vi "RegisterMap_ RegMap Sort.vi"(8 "error in (no error)":errorcluster, 10 "Register RegMap Data":string[][](array[string]), 11 "Register Data IN":T1[](array[typedef]) {"Base" format="%.0x"; "Item Count" format="%.0x"; "Value" format="%.0x"; "RegMap"."Mask" format="%.0x"; "Default" format="%.0x"; "Register" format="%.0x"}) -> (0 "error out":errorcluster, 3 "Register Data OUT":T1[](array[typedef]) {"Base" format="%.0x"; "Item Count" format="%.0x"; "Value" format="%.0x"; "RegMap"."Mask" format="%.0x"; "Default" format="%.0x"; "Register" format="%.0x"})   [LabVIEW 2010]
doc: "This VI sorts the RegMap data that was split into components and updates the Register Map array with the information.\n\nInputs:\nAMC Register Data IN - (cluster[]) array containing register map data\nRegister RegMap Data - (str[]) string array containing the register format for each register\nerror in - error input cluster\n\nOutputs:\nAMC Register Data OUT - (cluster[]) updated input array\nBit Count Verify Array - (U16) array displaying counted length of each register (should all be equal to the register length/size) (LOCAL only)\nAll Registers Equal Length? - (bool) TRUE = all registers are equal length (LOCAL only)\nerror out - error output cluster"
uses:
  TYP_ADSxxxx Register.ctl
  TYP_RegMap Item.ctl
panel:
  out "All Register Equal Length?":bool
  out "Bit Count Verify Array":u16[](array[numeric])
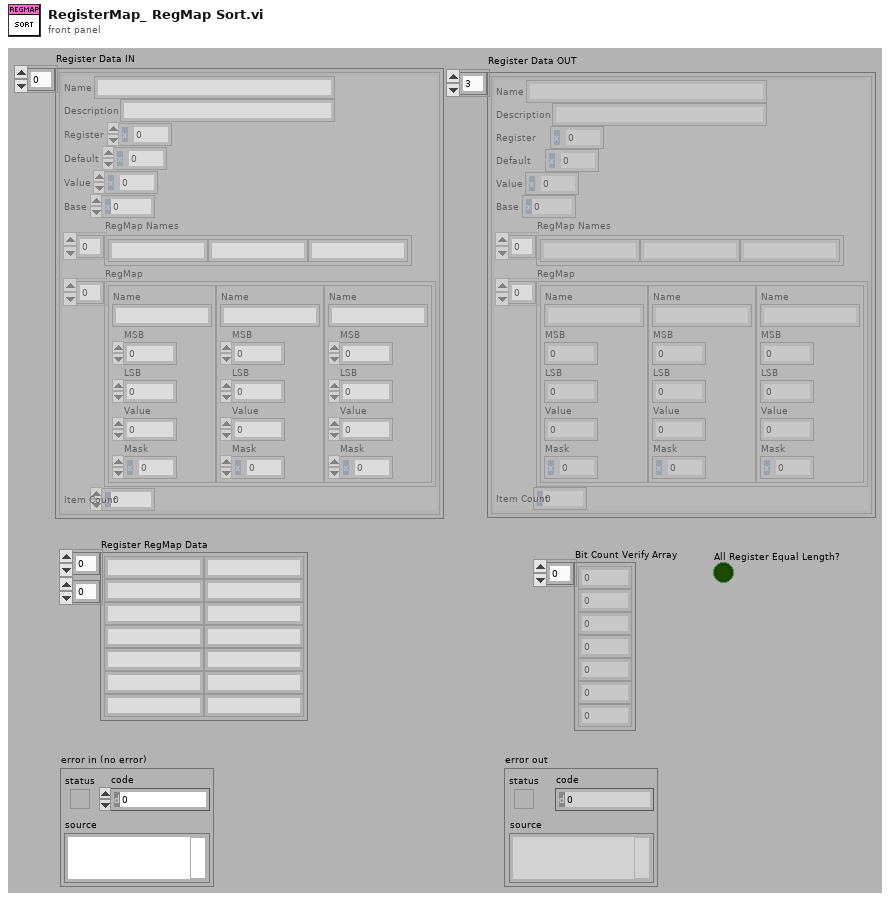
[diagram p1: front panel]
types:
  T1 = typedef "TYP_ADSxxxx Register.ctl" = cluster{"Name":string, "Description":string, "Register":u16, "Default":u16, "Value":u16, "Base":u16, "RegMap Names":string[], "RegMap":T2[], "Item Count":u8}
  T2 = typedef "TYP_RegMap Item.ctl" = cluster{"Name":string, "MSB":u16, "LSB":u16, "Value":u16, "Mask":u16}
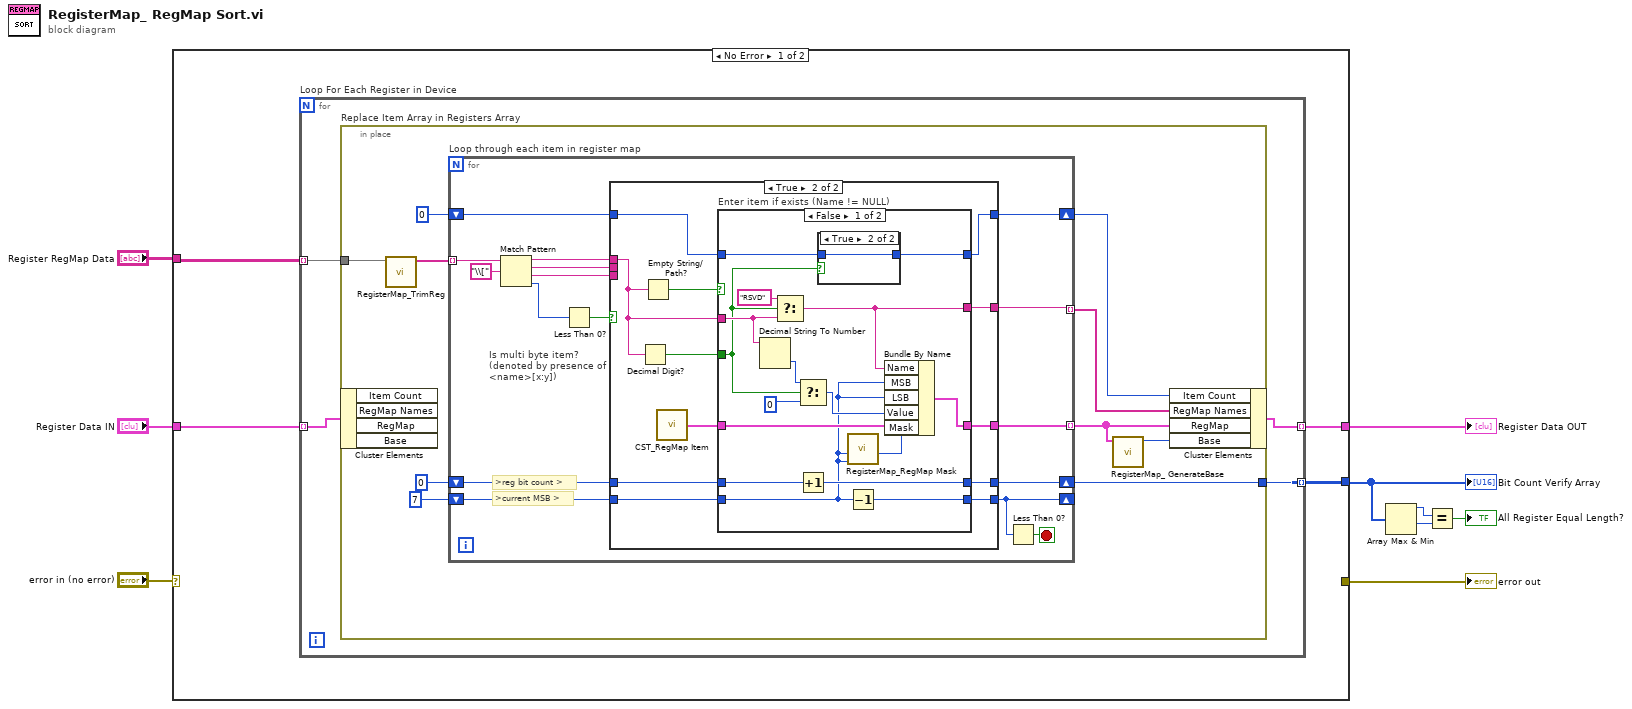
[diagram p0: block diagram]
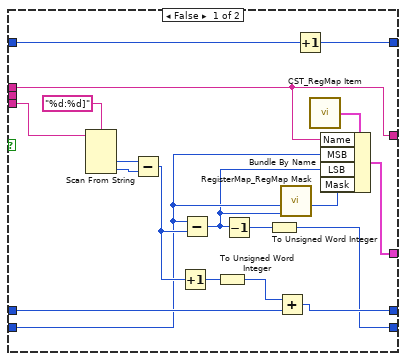
[diagram p2: hidden frame]
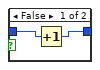
[diagram p3: hidden frame]
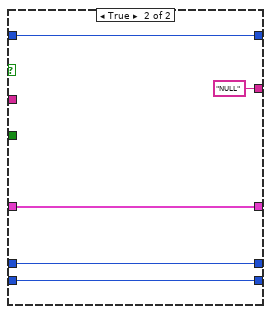
[diagram p4: hidden frame]
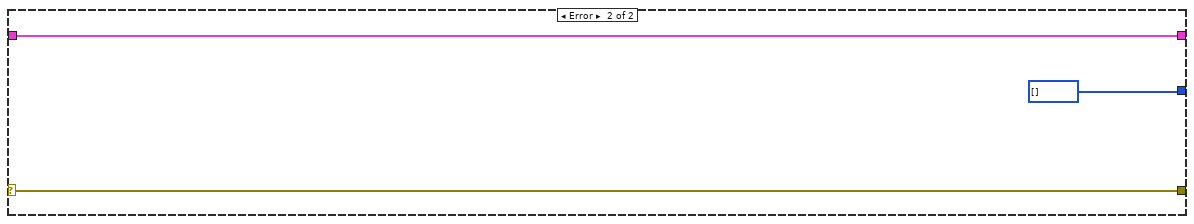
[diagram p5: hidden frame]
diagram:
  n1 = case shown="No Error" "error in (no error)" {
    selector: "error in (no error)" -> [_ w101]
    tunnel: "Register RegMap Data" -> [w11 _]
    tunnel: "Register Data IN" -> [w13 w100]
    tunnel: [w12 w100] -> w7
    tunnel: [_ w101] -> w5
    tunnel: [w10 u16[] []] -> w1
    frame No Error {
      n2 = for "Loop For Each Register in Device" {
        tunnel: w11 -> [w17] mode=indexing
        tunnel: [w16] -> w10 mode=indexing
        tunnel: w13 -> [w15] mode=indexing
        tunnel: [w14] -> w12 mode=indexing
        n3 = in-place "Replace Item Array in Registers Array" {
          in-place-border: w17 -> [w21]
          in-place-border: [w26] -> w16
          n4 = in-place-cluster #1(w15) -> ()  [unwired: 4 out]
          n5 = call "RegisterMap_TrimReg.vi"("Register RegMap Data IN"=w21) -> ("Register RegMap Data OUT"=w20:string[])  [unwired: 10 out]
          n6 = for "Loop through each item in register map" {
            tunnel: w20 -> [w43] mode=indexing
            shift-right: [w35] -> w26
            shift-left: u16 0 -> [w36]
            shift-right: [w30] -> _
            shift-left: u16 7 -> [w34]
            tunnel: [w33] -> w19 mode=indexing
            tunnel: [w32] -> w24 mode=indexing
            shift-right: [w28] -> w22
            shift-left: u8 0 -> [w29]
            stop <- w31 stop-if-true
            # ">current MSB >"
            # ">reg bit count >"
            n7 = Match Pattern(string=w43, regular expression="\\[") -> (before substring=w37:string, match substring=w38:string, after substring=w39:string, offset past match=w41:i32)  [unwired: 1 out]
            n8 = Less Than 0?(x=w41) -> (x < 0?=w40:bool)
            n9 = case "Is multi byte item?  (denoted by presence of <name>[x:y])" shown="True" w40 {
              tunnel: w39 -> [w57 _]
              tunnel: w38 -> [_ _]
              tunnel: w37 -> [w51 w67]
              tunnel: [w59 w74] -> w35
              tunnel: w36 -> [w58 w73]
              tunnel: w34 -> [w50 w70]
              tunnel: [w55 w71] -> w33
              tunnel: [w47 w69] -> w30
              tunnel: [w51 w65] -> w32
              tunnel: w29 -> [w45 w64]
              tunnel: [w44 w63] -> w28
              frame False {
                n10 = Scan From String(format string="%d:%d]", input string=w57) -> (output 1=w61:i32, output 2=w60:i32)  [unwired: 2 in, 5 out]
                n11 = Subtract(x=w61, y=w60) -> (x-y=w53:i32)
                n12 = Increment(x=w53) -> (x+1=w56:i32)
                n13 = Subtract(x=w50, y=w53) -> (x-y=w49:i32)
                n14 = To Unsigned Word Integer(number=w56) -> (unsigned 16bit integer=w46:u16)
                n15 = Decrement(x=w49) -> (x-1=w54:i32)
                n16 = To Unsigned Word Integer(number=w54) -> (unsigned 16bit integer=w47:u16)
                n17 = Add(x=w46, y=w58) -> (x+y=w59:u16)
                n18 = call "RegisterMap_RegMap Mask.vi"("LSB"=w49, "MSB"=w50) -> ("Mask"=w48:u16)  [unwired: 9 out]
                n19 = Increment(x=w45) -> (x+1=w44:u8)
                n20 = call "CST_RegMap Item.vi"() -> ("RegMap Item"=w52:T2)  [unwired: 1 out]
                n21 = Bundle By Name(cluster=w52, "Name"=w51, "MSB"=w50, "LSB"=w49, "Mask"=w48) -> (w55:T2)
              }
              frame True {
                n22 = Decimal Digit?(1:w67) -> (0:w68:bool)
                n23 = Empty String/Path?(string/path=w67) -> (empty?=w72:bool)
                n24 = call "CST_RegMap Item.vi"() -> ("RegMap Item"=w66:T2)  [unwired: 1 out]
                n25 = case "Enter item if exists (Name != NULL)" shown="False" w72 {
                  tunnel: [w89 w98] -> w74
                  tunnel: w73 -> [w87 w98]
                  tunnel: w66 -> [w90 w97]
                  tunnel: w67 -> [w83 _]
                  tunnel: [w88 w97] -> w71
                  tunnel: w70 -> [w80 w96]
                  tunnel: [w86 w96] -> w69
                  tunnel: w68 -> [w77 _]
                  tunnel: [w82 "NULL" ("token string")] -> w65
                  tunnel: w64 -> [w76 w94]
                  tunnel: [w75 w94] -> w63
                  frame False {
                    n26 = Decimal String To Number(string=w83) -> (number=w78:i32)  [unwired: 3 out]
                    n27 = Select(t="RSVD", s=w77, f=w83) -> (s? t:f=w82:string)
                    n28 = Select(t=w78, s=w77, f=0) -> (s? t:f=w84:i32)
                    n29 = Increment(x=w87) -> (x+1=w89:u16)
                    n30 = case shown="True" w77 {
                      tunnel: w76 -> [w91 w93]
                      tunnel: [w92 w93] -> w75
                      frame False {
                        n31 = Increment(x=w91) -> (x+1=w92:u8)
                      }
                      frame True {
                      }
                    }
                    n32 = call "RegisterMap_RegMap Mask.vi"("LSB"=w80, "MSB"=w80) -> ("Mask"=w81:u16)  [unwired: 9 out]
                    n33 = Decrement(x=w80) -> (x-1=w86:u16)
                    n34 = Bundle By Name(cluster=w90, "Name"=w82, "MSB"=w80, "LSB"=w80, "Value"=w84, "Mask"=w81) -> (w88:T2)
                  }
                  frame True {
                  }
                }
              }
            }
            n35 = Less Than 0?(x=w30) -> (x < 0?=w31:bool)
          }
          n36 = call "RegisterMap_ GenerateBase.vi"("RegMap"=w19) -> ("Base Value"=w18:u16)  [unwired: 10 in]
          n37 = in-place-cluster #1("Item Count"=w22, "RegMap Names"=w24, "RegMap"=w19, "Base"=w18) -> (w14:T1)
        }
      }
    }
    frame Error {
    }
  }
  "Bit Count Verify Array" <- w1
  "Register Data OUT" <- w7
  "error out" <- w5
  n38 = Array Max & Min(array=w1) -> (max value=w3:u16, min value=w4:u16)  [unwired: 2 out]
  n39 = Equal?(x=w3, y=w4) -> (x = y?=→"All Register Equal Length?":bool)
